vi "Constant_Thermal_Efficiency_Check.vi"(10 "Totalized Flow (Gallons)":string, 11 "Totalizer [Sft3]":string) -> (2 "Constant Thermal Efficiency?":bool, 3 "Totalizer [Sft3]":dbl)   [LabVIEW 2023]
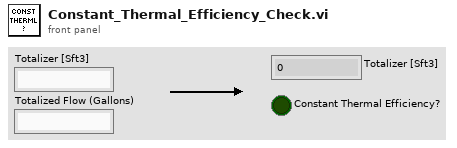
[diagram p1: front panel]
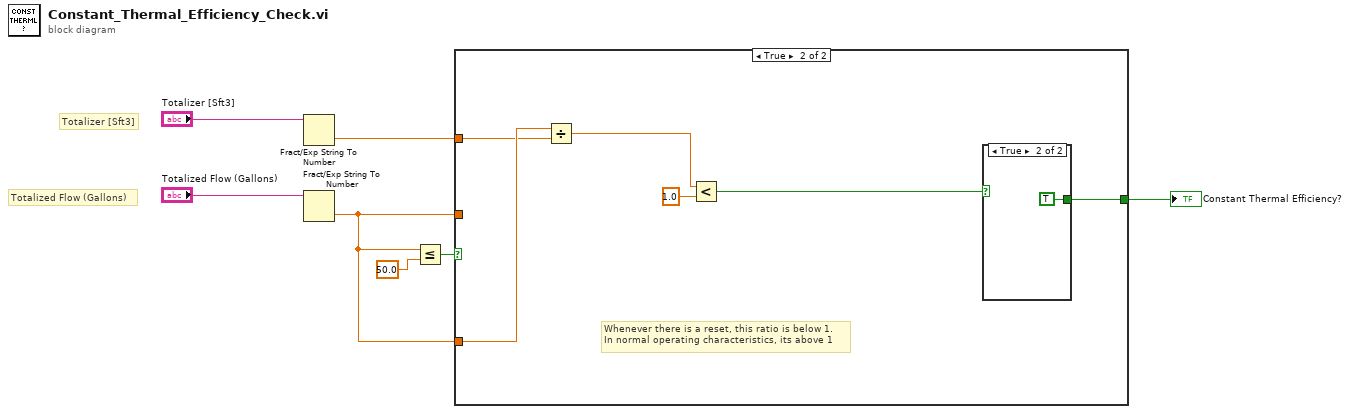
[diagram p0: block diagram]
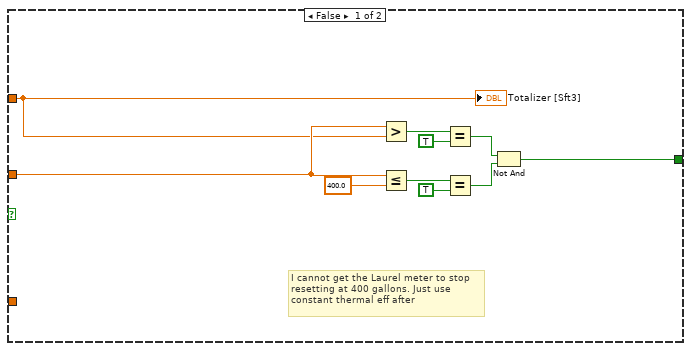
[diagram p2: hidden frame]
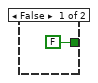
[diagram p3: hidden frame]
diagram:
  # "Totalizer [Sft3]"
  # "Totalized Flow (Gallons)"
  n1 = Fract/Exp String To Number(string="Totalizer [Sft3]") -> (number=w2:dbl)  [unwired: 3 in, 1 out]
  n2 = Fract/Exp String To Number(string="Totalized Flow (Gallons)") -> (number=w1:dbl)  [unwired: 3 in, 1 out]
  n3 = Less Or Equal?(x=w1, y=50.0) -> (x <= y?=w4:bool)
  n4 = case shown="True" w4 {
    tunnel: [w9 w23] -> w6
    tunnel: w1 -> [w16 _]
    tunnel: w2 -> [w8 w21]
    tunnel: w1 -> [_ w22]
    frame False {
      # "I cannot get the Laurel meter to stop\nresetting at 400 gallons. Just use \nconstant thermal eff after"
      n5 = Greater?(x=w16, y=w8) -> (0:w15:bool)
      n6 = Less Or Equal?(x=w16, y=400.0) -> (x <= y?=w13:bool)
      n7 = Equal?(x=w15, y=TRUE) -> (x = y?=w11:bool)
      n8 = Equal?(x=w13, y=TRUE) -> (x = y?=w10:bool)
      n9 = Not And(1:w10, 2:w11) -> (0:w9:bool)
      "Totalizer [Sft3]" <- w8
    }
    frame True {
      # "Whenever there is a reset, this ratio is below 1.\nIn normal operating characteristics, its above 1"
      n10 = Divide(x=w22, y=w21) -> (x/y=w18:dbl)
      n11 = Less?(x=w18, y=1.0) -> (x < y?=w19:bool)
      n12 = case shown="True" w19 {
        tunnel: [FALSE TRUE] -> w23
        frame False {
        }
        frame True {
        }
      }
    }
  }
  "Constant Thermal Efficiency?" <- w6
